vi "OscilloscopeSettings.vi"(8 "error in (no error)":errorcluster, 10 "Settings cluster":T2 {"MeasureMode" items=["Block"=2, "Stream"=1]; "Bitness" items=["16 bit"=16, "14 bit"=14, "12 bit"=12]}, 11 "hDevice in":u32) -> (0 "error out":errorcluster, 2 "Actual settings":T1, 3 "hDevice out":u32)   [LabVIEW 2018]
uses:
  LibTiePie.lvlib
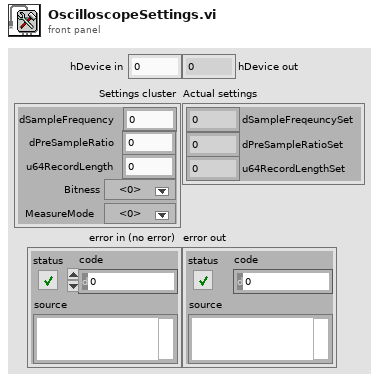
[diagram p1: front panel]
types:
  T1 = cluster{"u64RecordLengthSet":u64, "dPreSampleRatioSet":dbl, "dSampleFreqeuncySet":dbl}
  T2 = cluster{"u64RecordLength":u64, "dPreSampleRatio":dbl, "dSampleFrequency":dbl, "MeasureMode":u32, "Bitness":u8}
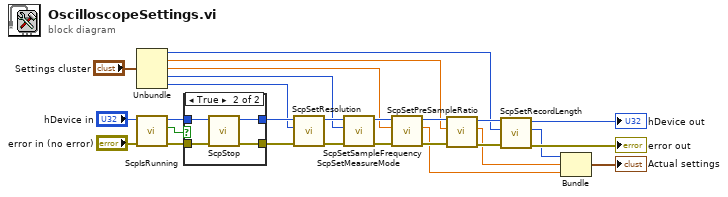
[diagram p0: block diagram]
diagram:
  n1 = Unbundle("Settings cluster") -> ("u64RecordLength"=w7:u64, "dPreSampleRatio"=w6:dbl, "dSampleFrequency"=w8:dbl, "MeasureMode"=w9:u32, "Bitness"=w10:u8)
  n2 = call "ScpIsRunning.vi"("error in (no error)"="error in (no error)", "hDevice in"="hDevice in") -> ("error out"=w26:errorcluster, "IsRunning?"=w25:bool, "hDevice out"=w27:u32)  [unwired: 7 in]
  n3 = case shown="True" w25 {
    tunnel: w27 -> [w28 w33]
    tunnel: w26 -> [w29 w32]
    tunnel: [w29 w30] -> w23
    tunnel: [w28 w31] -> w24
    frame False {
    }
    frame True {
      n4 = call "ScpStop.vi"("error in (no error)"=w32, "hDevice in"=w33) -> ("error out"=w30:errorcluster, "hDevice"=w31:u32)  [unwired: 7 in, 1 out]
    }
  }
  n5 = call "ScpSetResolution.vi"("error in (no error)"=w23, "byResolution"=w10, "hDevice in"=w24) -> ("error out"=w22:errorcluster, "hDevice out"=w21:u32)  [unwired: 6 in, 1 out]
  n6 = call "ScpSetMeasureMode.vi"("error in (no error)"=w22, "MeasureMode"=w9, "hDevice in"=w21) -> ("error out"=w19:errorcluster, "hDevice out"=w20:u32)  [unwired: 6 in, 1 out]
  n7 = call "ScpSetSampleFrequency.vi"("error in (no error)"=w19, "dSampleFrequency"=w8, "hDevice in"=w20) -> ("error out"=w17:errorcluster, "dSampleFreqeuncySet"=w3:dbl, "hDevice out"=w18:u32)  [unwired: 6 in]
  n8 = call "ScpSetPreSampleRatio.vi"("error in (no error)"=w17, "dPreSampleRatio in"=w6, "hDevice in"=w18) -> ("error out"=w16:errorcluster, "dPreSampleRatioSet"=w4:dbl, "hDevice out"=w15:u32)  [unwired: 6 in]
  n9 = call "ScpSetRecordLength.vi"("error in (no error)"=w16, "u64RecordLength"=w7, "hDevice in"=w15) -> ("error out"=→"error out":errorcluster, "u64RecordLengthSet"=w5:u64, "hDevice out"=→"hDevice out":u32)  [unwired: 6 in]
  n10 = Bundle("u64RecordLengthSet"=w5, "dPreSampleRatioSet"=w4, "dSampleFreqeuncySet"=w3) -> (→"Actual settings":T1)  [unwired: 1 in]
